vi "실습2-4텍스트링.vi"() -> ()   [LabVIEW 2014]
panel:
  out "초 단위":dbl=120.0
  in  "시간입력 2":dbl=2.0
  in  "링":u32(ring)=60 items=["일"=86400, "시간"=3600, "분"=60, "초"=1]
  out "타임스탬프":timestamp
  out "색 상자":u32(colorbox)
  in  "숫자형":u32 format="%.0x"
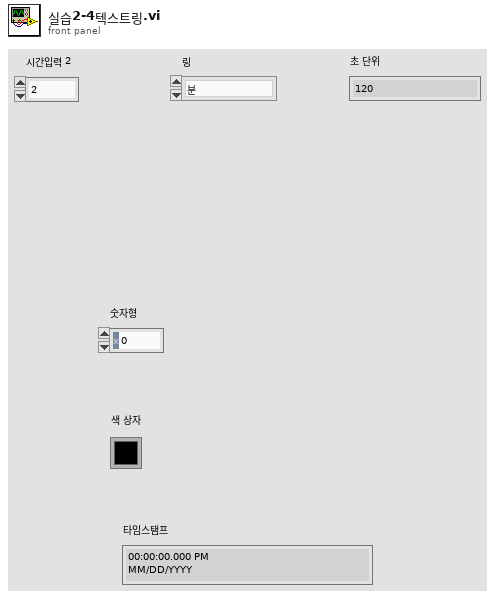
[diagram p1: front panel]
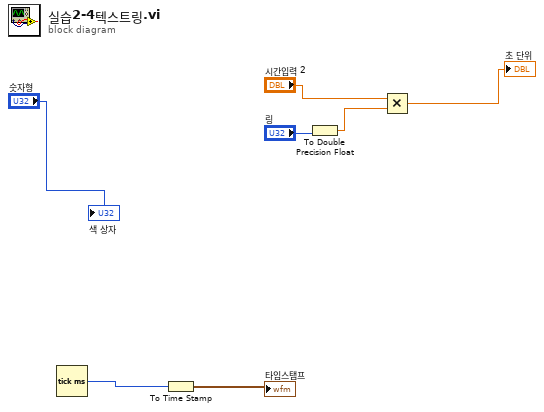
[diagram p0: block diagram]
diagram:
  n1 = Tick Count (ms)() -> (millisecond timer value=w2:u32)
  n2 = To Time Stamp(1:w2) -> (0:→"타임스탬프":timestamp)
  n3 = To Double Precision Float(number="링") -> (double precision float=w4:dbl)
  n4 = Multiply(x="시간입력 2", y=w4) -> (x*y=→"초 단위":dbl)
  "색 상자" <- "숫자형"
